vi "baogao1.vi"() -> ()   [LabVIEW 2017]
panel:
  out "y":i32[](array[numeric])
  out "x":i32
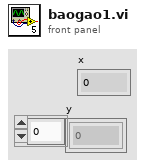
[diagram p1: front panel]
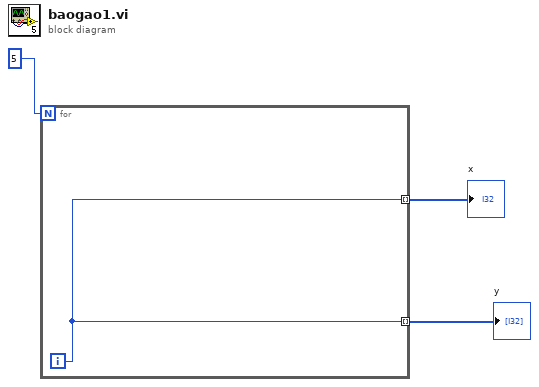
[diagram p0: block diagram]
diagram:
  n1 = for {
    N: 5 -> [_]
    tunnel: [w4] -> w1 mode=indexing
    tunnel: [w4] -> w2 mode=indexing
    i -> [w4]
  }
  "x" <- w1
  "y" <- w2
